vi "Blink.vi"(11 "Blink_Rate (hz)":i32) -> (3 "Blink":bool)   [LabVIEW 2018, in "ArgoBotLib.lvlib"]
uses:
  ArgoBotLib.lvlib
panel:
  # "Blink at a constant Hz"
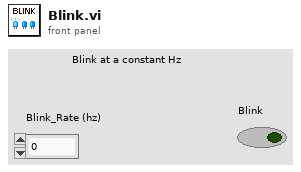
[diagram p1: front panel]
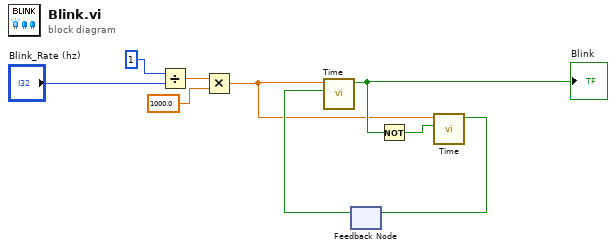
[diagram p0: block diagram]
diagram:
  n1 = Divide(x=1, y="Blink_Rate (hz)") -> (x/y=w3:dbl)
  n2 = Multiply(x=w3, y=1000.0) -> (x*y=w1:dbl)
  n3 = feedback #1() -> (w9:bool)  [unwired: 1 in]
  n4 = call "Time.vi"("Reset"=w9, "Time_Limit"=w1) -> ("Time_Met"=w8:bool)  [unwired: 9 in]
  "Blink" <- w8
  n5 = Not(x=w8) -> (.not. x?=w7:bool)
  n6 = call "Time.vi"("Reset"=w7, "Time_Limit"=w1) -> ("Time_Met"=w6:bool)  [unwired: 9 in]
  n7 = feedback-in #1(w6) -> ()
